vi "Define_Original_Problem_Point_in_Subtrack-1.vi"(4 "[IN] Statuses":i16[](array[numeric])) -> (0 "[OUT] Index of Displace\nment Before or After":i32, 2 "[OUT] Index of Problem Point\nin Subtrack (Original)":i32)   [LabVIEW 2013]
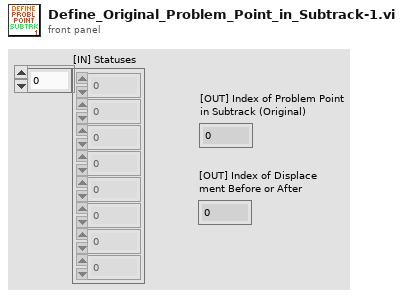
[diagram p1: front panel]
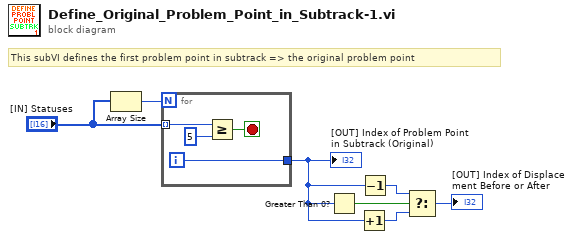
[diagram p0: block diagram]
diagram:
  # "This subVI defines the first problem point in subtrack => the original problem point"
  n1 = Array Size(array="[IN] Statuses") -> (size(s)=w7:i32)
  n2 = for {
    N: w7 -> [_]
    tunnel: "[IN] Statuses" -> [w11] mode=indexing
    tunnel: [w8] -> w3
    i -> [w8]
    stop <- w9 stop-if-true
    n3 = Greater Or Equal?(x=w11, y=i16 5) -> (x >= y?=w9:bool)
  }
  "[OUT] Index of Problem Point\nin Subtrack (Original)" <- w3
  n4 = Greater Than 0?(x=w3) -> (x > 0?=w5:bool)
  n5 = Increment(x=w3) -> (x+1=w2:i32)
  n6 = Decrement(x=w3) -> (x-1=w4:i32)
  n7 = Select(t=w4, s=w5, f=w2) -> (s? t:f=→"[OUT] Index of Displace\nment Before or After":i32)
